vi "Write Camera.vi"(7 "error in (no error)":errorcluster, 9 "Camera":T1, 10 "Gantry Class in":refnum<class "Gantry Class.lvclass">) -> (0 "error out":errorcluster, 3 "Gantry Class out":refnum<class "Gantry Class.lvclass">)   [LabVIEW 2011, in "Gantry Class.lvclass"]
uses:
  Gantry Class.lvclass
  Type Definitions/Gantry_Camera.ctl
  <vilib>/userDefined/High Color/IMAQdx.ctl
  Gantry Class.lvclass/Gantry Class.ctl
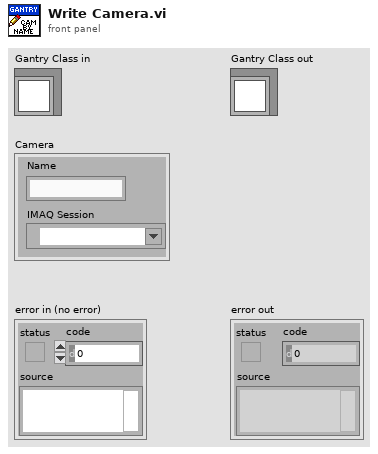
[diagram p1: front panel]
types:
  T1 = typedef "Gantry_Camera.ctl" = cluster{"Name":string, "IMAQ Session":T2}
  T2 = typedef "IMAQdx.ctl" = refnum<k21>
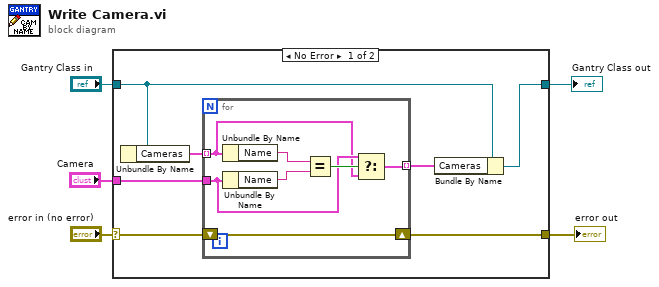
[diagram p0: block diagram]
diagram:
  n1 = case shown="No Error" "error in (no error)" {
    selector: "error in (no error)" -> [w11 w20]
    tunnel: [w10 w20] -> w4
    tunnel: [w7 w21] -> w2
    tunnel: "Gantry Class in" -> [w8 w21]
    tunnel: "Camera" -> [w9 _]
    frame No Error {
      n2 = Unbundle By Name(w8) -> ("Cameras"=w12:T1[])
      n3 = for {
        tunnel: w12 -> [w13] mode=indexing
        shift-right: [w19] -> w10
        shift-left: w11 -> [w19]
        tunnel: w9 -> [w15]
        tunnel: [w14] -> w6 mode=indexing
        n4 = Unbundle By Name(w13) -> ("Name"=w17:string)
        n5 = Unbundle By Name(w15) -> ("Name"=w18:string)
        n6 = Equal?(x=w17, y=w18) -> (x = y?=w16:bool)
        n7 = Select(t=w15, s=w16, f=w13) -> (s? t:f=w14:T1)
      }
      n8 = Bundle By Name(cluster=w8, "Cameras"=w6) -> (w7:refnum<class "Gantry Class.lvclass">)
    }
    frame Error {
    }
  }
  "error out" <- w4
  "Gantry Class out" <- w2
